vi "MM6Archiver.change file.vi"(0 "i ref in":refnum<vi>, 3 "ms timeout (10000)":i32=10000, 5 "error in (no error)":errorcluster) -> (14 "i ref out":refnum<vi>, 17 "timed out":bool, 19 "error out":errorcluster)   [LabVIEW 2014, in "MM6Archiver.lvlib"]
doc: "Overwrite method. No action performed, since MM6 archiver does not support files names with numbers incremented."
uses:
  MM6Archiver.lvlib
  CS_Core/CSSystem/CoreDefs/CoreDefs.rawDataType.ctl
  CSData/DiscArchiver/DiscArchiver.lvlib
  CSData/DataLib/DataLib.lvlib
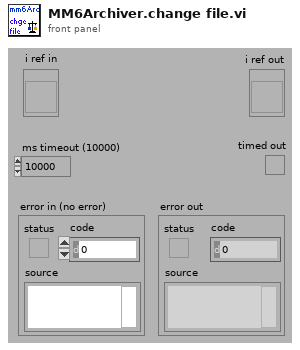
[diagram p1: front panel]
types:
  T1 = typedef "CoreDefs.rawDataType.ctl" = i8[]
  T2 = typedef "DiscArchiver.lvlib/DiscArchiver.i attribute.ctl" = cluster{"file prefix":string, "actual file":string, "nOfEvents":i32, "file":refnum<file>, "eventBuilder":string, "disc size alarm":bool, "dataDescription":string, "dataDescriptionURL":string, "eventDataURL":string, "headerID":dbl, "completeData":bool, "nOfEventsID":i32, "dataFileID":i32}
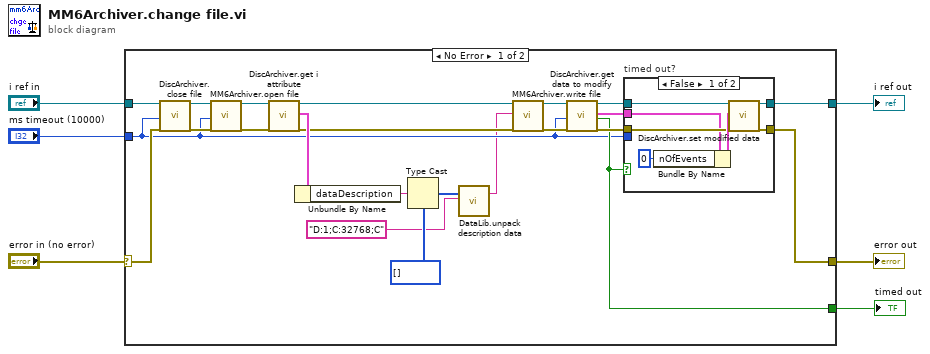
[diagram p0: block diagram]
diagram:
  n1 = case shown="No Error" "error in (no error)" {
    selector: "error in (no error)" -> [w16 w39]
    tunnel: [w29 w40] -> w3
    tunnel: "i ref in" -> [w25 w40]
    tunnel: "ms timeout (10000)" -> [w12 _]
    tunnel: [w17 w39] -> w2
    tunnel: [w15 _] -> w1
    frame No Error {
      n2 = call "DiscArchiver.close file.vi"("i ref in"=w25, "ms timeout (10000)"=w12, "error in (no error)"=w16) -> ("i ref out"=w24:refnum<vi>, "error out"=w23:errorcluster)  [unwired: 14 in, 1 out]
      n3 = call "MM6Archiver.open file.vi"("i ref in"=w24, "ms timeout (10000)"=w12, "error in (no error)"=w23) -> ("i ref out"=w22:refnum<vi>, "error out"=w21:errorcluster)  [unwired: 14 in, 1 out]
      n4 = call "DiscArchiver.get i attribute.vi"("i ref in"=w22, "error in (no error)"=w21) -> ("i ref out"=w14:refnum<vi>, "i attribute"=w20:T2, "error out"=w13:errorcluster)  [unwired: 15 in]
      n5 = Unbundle By Name(w20) -> ("dataDescription"=w11:string)
      n6 = Type Cast(type=T1 [] ("Array"), x=w11) -> (*(type *) &x=w9:T1)
      n7 = call "DataLib.unpack description data.vi"("serviceData"=w9, "descriptor"="D:1;C:32768;C") -> ("header"=w7:string)  [unwired: 14 in, 3 out]
      n8 = call "MM6Archiver.write file.vi"("i ref in"=w14, "eventData"=w7, "error in (no error)"=w13) -> ("i ref out"=w19:refnum<vi>, "error out"=w18:errorcluster)  [unwired: 15 in]
      n9 = call "DiscArchiver.get data to modify.vi"("i ref in"=w19, "ms timeout (10000)"=w12, "error in (no error)"=w18) -> ("i ref out"=w28:refnum<vi>, "i attribute"=w26:T2, "timed out"=w15:bool, "error out"=w27:errorcluster)  [unwired: 13 in]
      n10 = case "timed out?" shown="False" w15 {
        tunnel: [w36 w37] -> w17
        tunnel: [w35 w38] -> w29
        tunnel: w28 -> [w33 w38]
        tunnel: w27 -> [w31 w37]
        tunnel: w26 -> [w30 _]
        tunnel: w12 -> [_ _]
        frame False {
          n11 = Bundle By Name(cluster=w30, "nOfEvents"=0 ("# of items")) -> (w34:T2)
          n12 = call "DiscArchiver.set modified data.vi"("i ref in"=w33, "i attribute"=w34, "error in (no error)"=w31) -> ("i ref out"=w35:refnum<vi>, "error out"=w36:errorcluster)  [unwired: 15 in]
        }
        frame True {
        }
      }
    }
    frame Error {
    }
  }
  "error out" <- w2
  "i ref out" <- w3
  "timed out" <- w1
